vi "Show Animated Busy Icon.vi"(2 "Error In":errorcluster) -> (7 "Error Out":errorcluster)   [LabVIEW 2021, in "GUI.lvlib"]
doc: "This VI uses error in normally (doesn't do anything if there is an error in) and passes through the error in (ignores additional unternal errors)."
uses:
  GUI/GUI.lvlib
  Error/Error.lvlib
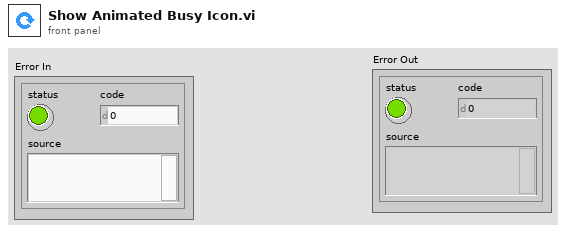
[diagram p1: front panel]
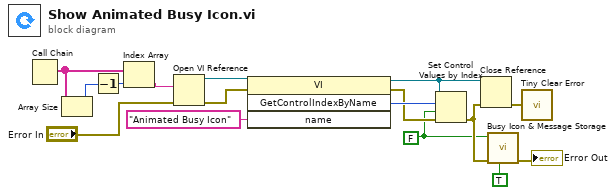
[diagram p0: block diagram]
diagram:
  w1 = FALSE ("Visible")
  n1 = Call Chain() -> (call chain=w16:string[])
  n2 = Array Size(array=w16) -> (size(s)=w15:i32)
  n3 = Decrement(x=w15) -> (x-1=w14:i32)
  n4 = Index Array(array=w16, index=w14) -> (element=w13:string)
  n5 = Open VI Reference(vi path=w13, error in (no error)="Error In") -> (vi reference=w8:refnum<vi>, error out=w9:errorcluster)  [unwired: 4 in]
  n6 = invoke class="VI" method="GetControlIndexByName"(reference=w8, error in=w9, "name"="Animated Busy Icon" ("element")) -> (reference out=w7:refnum<vi>, error out=w10:errorcluster, "GetControlIndexByName"=w11:i32)  [unwired: 1 in, 1 out]
  n7 = Set Control Values by Index(0:w7, 1:w11, 2:w1, 3:w10) -> (11:w4:errorcluster)
  n8 = Close Reference(reference=w7, error in (no error)=w4) -> (error out=w5:errorcluster)
  n9 = call "Busy Icon & Message Storage.vi"("Get(F)/Set Busy Icon"=TRUE, "Error In"=w4, "Busy Icon Status (F = busy)"=w1) -> ("Error Out"=→"Error Out":errorcluster)  [unwired: 6 in, 2 out]
  n10 = call "Tiny Clear Error.vi"("Error In"=w5) -> ()  [unwired: 8 in, 1 out]
